vi "5ChPulserTrigs.vi"(1 "Motion Board ID":T3=1 min=1 max=32 step=1, 4 "xmit ring":i32 min=0 max=4 step=1, 5 "mode":T2=enum."Full 25 Ch", 6 "Source":tag="/Dev1/PFI9" caption="Trigger Source", 7 "high time":dbl=5e-06 format="%^.2e", 8 "Axis":T1=1 caption="Axis or Vector Space" items=["Axis 1"=1, "Axis 2"=2, "Axis 3"=3, "Axis 4"=4, "Axis 5"=5, "Axis 6"=6, "Axis 7"=7, "Axis 8"=8, "Vector Space 1"=17, "Vector Space 2"=18, "Vector Space 3"=19, "Vector Space 4"=20], 9 "M-mode?":bool, 10 "error in":errorcluster) -> (0 "5CH Pulser Tasks":refnum<k21>[](array[refnum]), 3 "error out":errorcluster)   [LabVIEW 2022 SP3]
uses:
  ScanningControl/Motion Controllers/-MotionRoutines/MotionGlobals.vi
  <vilib>/DAQmx/configure/trigger.llb/DAQmx Start Trigger (Digital Edge).vi
  <vilib>/DAQmx/create/channels.llb/DAQmx Create Channel (CO-Pulse Generation-Time).vi
  <resource>/objmgr/daqmx.rc
  <vilib>/DAQmx/create/channels.llb/DAQmx Create Channel (CO-Pulse Generation-Frequency).vi
  <vilib>/DAQmx/configure/timing.llb/DAQmx Timing (Implicit).vi
  ScanningControl/Digitizers/-DigitizerRoutines/DigitizerGlobals.vi
  ScanningControl/Switch Modules/SwitchGlobals.vi
  Real Time/-RT_support/RealTimeMode.ctl
  <vilib>/Motion/FlexMotion/CustomControls/CustomControls.llb/AxisOrVectorSpace To Control.flx
panel:
  in  "stop":bool
  # "Counter 1 output is the BNC on grey box."
  # "Trigger source comes from Gate of CTR0 (PFI9)\n\nThe NI trigger connector routes to CTR0 Gate"
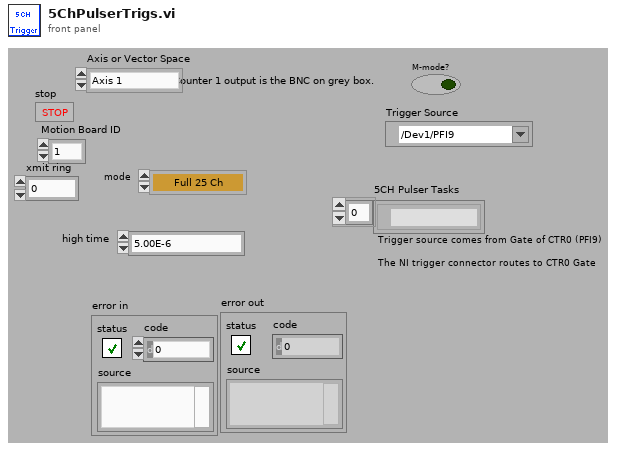
[diagram p1: front panel]
types:
  T1 = typedef "AxisOrVectorSpace To Control.flx" = u16
  T2 = typedef "RealTimeMode.ctl" = enum16{"1T/5R", "1T/5R Deep Mem", "Full 25 Ch", "Drop Ch 5", "Drop Ch 5,4", "Drop Ch 5,4,3", "Drop Ch 5,4,3,2", "All 25 FIFO CH by CH", "Line by line 2 Ch", "Line by line All", "Deep Memory 2 CH", "Drop Ch 5 (3 Trig)", "test", "Drop Ch 5 XMIT", "Drop Ch 5,4 XMIT", "Drop Ch 5,4,3 XMIT"}
  T3 = typedef "Board Id" = u8
  T4 = typedef "DigitizerSettings.ctl" = cluster{"Digitizer delay (us) ":dbl, "rf points per line":i32, "lines per plane":i32, "Samp Rate (Hz)":dbl, "Additional dig delay (us)":dbl, "Voltage Scale":dbl, "Pre-Looks":i32, "Offset delay (us)":dbl, "bits A/D":i8, "Avg Num":i32, "DigTimeOut":sgl, "Rel Dig Delay":sgl, "Dig Ch":i32, "LeCroyCluster":cluster{"LeCroy Channels":bool[], "LC read pt offset":dbl, "Sweep Avg":bool}, "Main Digitizer":T5, "Dig Config":T6, "Digitizer ID Cluster":T7, "Trigger Settings":cluster{"Trig Source":u16, "Trig Coupling":u16, "Trig Slope":u16, "Level (mV)":dbl}, "Bulk Acq":bool, "Bulk Start Indexes":i32[], "Data Ref RF":refnum<data-value>, "NI ID/Channel":cluster{"NI ID":refnum<k15>, "NI CH":i32}[], "Total Dig CH":i32, "Xtra Ann Trig delay (us)":dbl, "Fix Z Delay?":bool, "One Way Transmission?":bool, "Data Ref Log":refnum<data-value>}
  T5 = typedef "Digitizer.ctl" = enum16{"Acqiris Digitizer", "NI Digitizer", "LeCroy", "GaGe", "AlazarTech", "No Digitizer", "Teledyne"}
  T6 = typedef "DigConfig.ctl" = enum16{"Single channel", "2 Chans w/ 2 Acqiris", "2 Chans w/ 1 Acqiris", "5-CH Pulser New", "5-CH pulser w/ ann array", "5-pass style ann array", "Empty"}
  T7 = typedef "DigitizerID.ctl" = cluster{"Acqiris/Alazar/SP ID":u32[], "NI Instr Handles":refnum<k15>[], "LeCroy VISA":refnum<visa-resource-name>, "GaGe Handle":cluster{"Handle":u32, "Sample size":u32, "Resolution":i32, "Offset":i32, "Channels":u32, "Boards":u32}, "ATS Ref":string, "Acqiris Address":string[], "ADQRef":refnum<k24>, "adq_cu_ptr":refnum<k24>}
  T8 = typedef "MotionParameters.ctl" = cluster{"No Motion?":bool, "Motion System":T9, "Motion Bd ID":u8, "Motion Profile":string, "# Axis":i8, "Reverse Z axis?":bool, "SMAC Axis":u16, "scan pair":T10, "RT fps":sgl, "Steps per mm":i32[], "Motor Parameters":cluster{"velocity ct/s":dbl[], "accel ct/s^2":dbl[]}, "One Way Scan":bool, "Reverse One Way Scan":bool, "Global Position (mm)":dbl[], "Plane":i32, "Distance between\nscan lines (um)":sgl, "Distance between\nscan planes (um)":sgl, "number of scan planes":i32, "Total steps in line":i32, "Xtra plane\ndistance  (um)":i32, "Xtra planes ":i32, "Add Axis":bool, "overshoot cts":i32, "BKPT Shift":i32, "Scan Start Time (ms)":u32, "ESP VISA":refnum<visa-resource-name>, "3rd Axis":T11, "GL Ref Out":refnum<k7>, "Galil Address":string}
  T9 = typedef "MotionSys.ctl" = enum16{"MM3000", "NI 735x", "Newport ESP", "No Motion Card", "Galil"}
  T10 = typedef "ScanAxis.ctl" = enum16{"y-(x) scan", "x-(y) scan", "z-(x) scan", "z-(y) scan", "y-(z) scan", "x-(z) scan", "w-(x) scan", "w-(y) scan", "w-(z) scan", "x-(w) scan", "y-(w) scan", "z-(w) scan"}
  T11 = typedef "3rdAxis.ctl" = u16
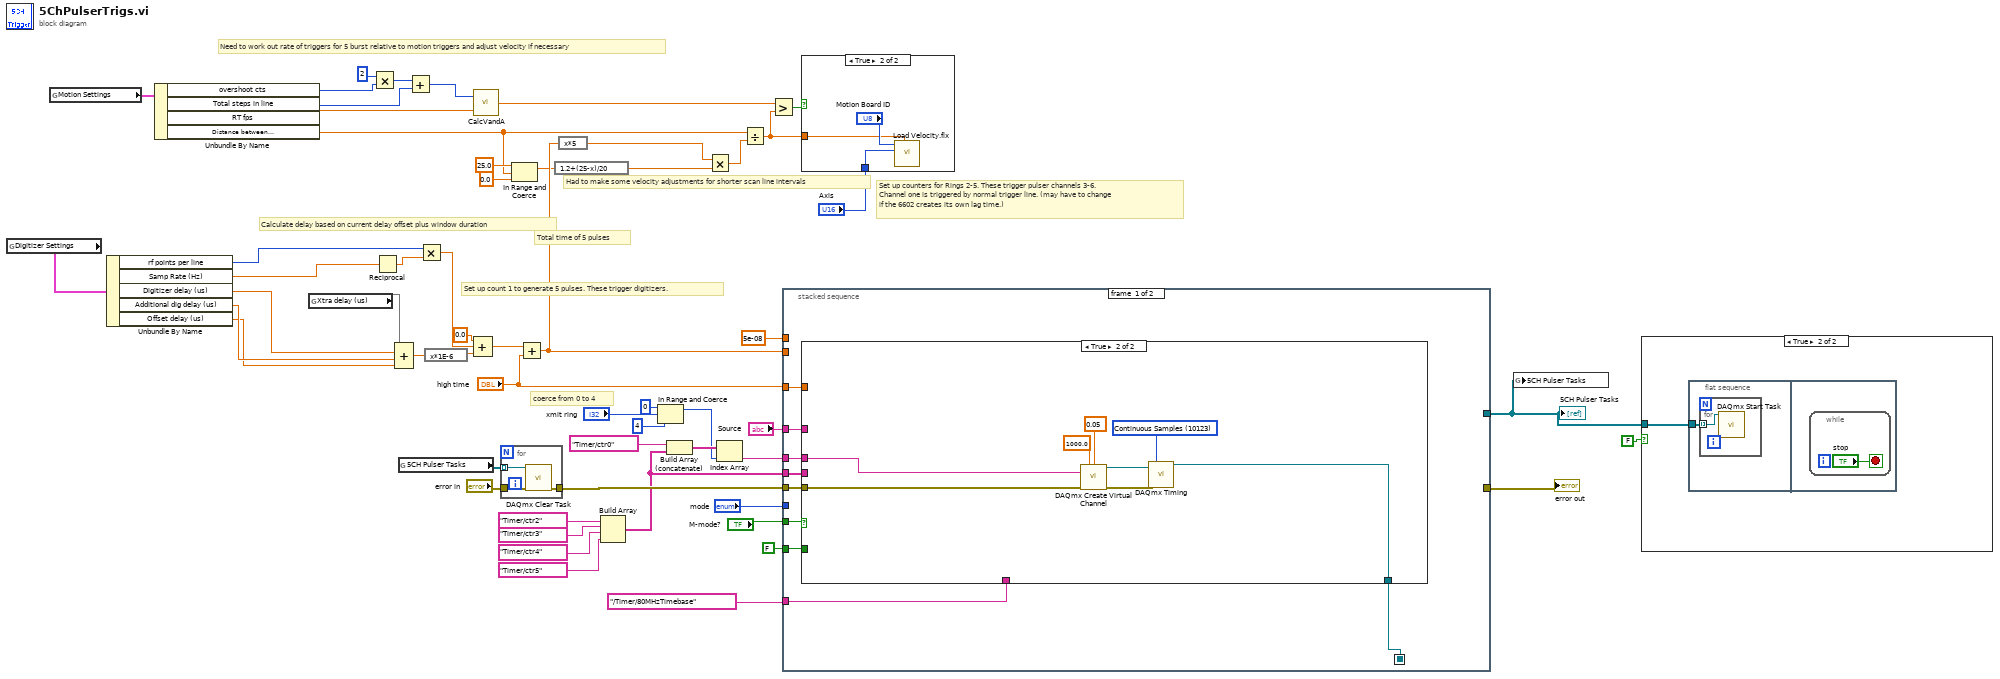
[diagram p0: block diagram]
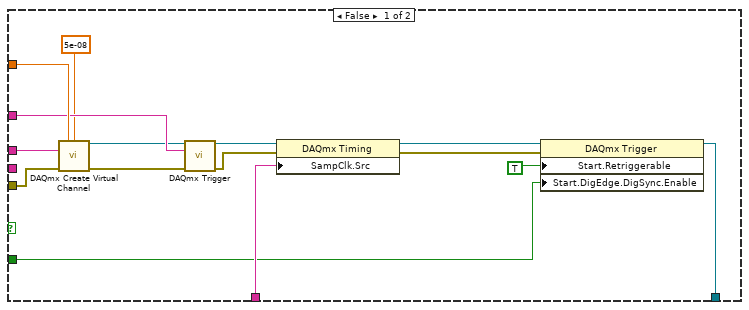
[diagram p2: hidden frame]
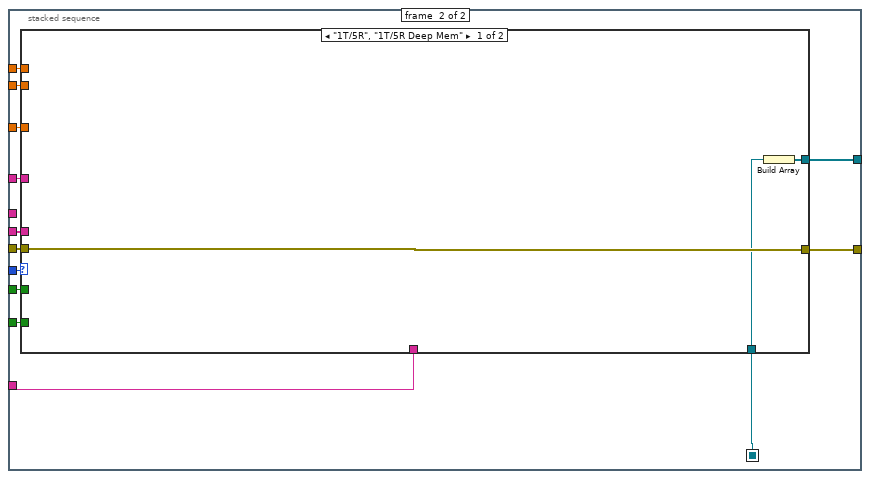
[diagram p3: hidden frame]
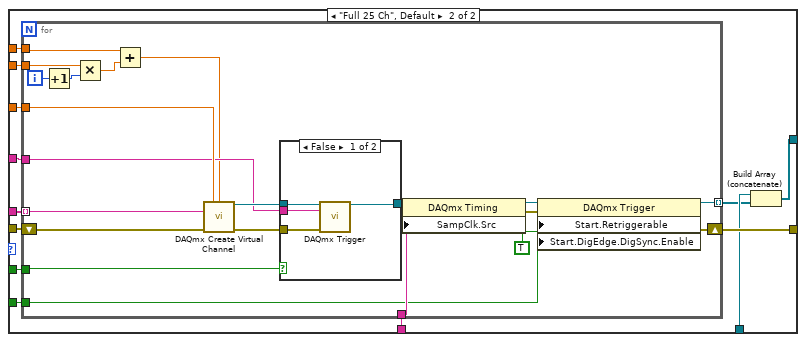
[diagram p4: hidden frame]
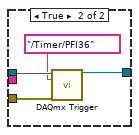
[diagram p5: hidden frame]
diagram:
  # "coerce from 0 to 4"
  # "Had to make some velocity adjustments for shorter scan line intervals"
  # "Total time of 5 pulses"
  # "Need to work out rate of triggers for 5 burst relative to motion triggers and adjust velocity if necessary"
  # "Set up counters for Rings 2-5. These trigger pulser channels 3-6.\nChannel one is triggered by normal trigger line. (may have to change \nif the 6602 creates its own lag time.)"
  # "Set up count 1 to generate 5 pulses. These trigger digitizers."
  # "Calculate delay based on current delay offset plus window duration"
  n1 = global read "DigitizerGlobals.vi" "Digitizer Settings"() -> (w7:T4)
  n2 = global read "MotionGlobals.vi" "Motion Settings"() -> (w12:T8)
  n3 = Unbundle By Name(w7) -> ("rf points per line"=w6:i32, "Samp Rate (Hz)"=w5:dbl, "Digitizer delay (us)"=w3:dbl, "Additional dig delay (us)"=w2:dbl, "Offset delay (us)"=w1:dbl)
  n4 = Unbundle By Name(w12) -> ("overshoot cts"=w11:i32, "Total steps in line"=w10:i32, "RT fps"=w9:sgl, "Distance between\nscan lines (um)"=w8:sgl)
  n5 = global read "SwitchGlobals.vi" "Xtra delay (us)"() -> (w4)
  n6 = Multiply(x=2, y=w11) -> (x*y=w45:i32)
  n7 = Reciprocal(x=w5) -> (1/x=w56:dbl)
  n8 = Compound Arithmetic op=ADD(w4, w3, w2, w1) -> (w29:dbl)
  n9 = global read "MotionGlobals.vi" "5CH Pulser Tasks"() -> (w51:refnum<k21>[])
  n10 = Add(x=w45, y=w10) -> (x+y=w44:i32)
  n11 = Multiply(x=w6, y=w56) -> (x*y=w57:dbl)
  n12 = expression code="x*1E-6"(w29) -> (w28:dbl)
  n13 = call "CalcVandA.vi"("distance"=w44, "fps"=w9) -> ("Velocity"=w42:dbl)  [unwired: 2 out]
  n14 = Compound Arithmetic op=ADD(0.0 ("y"), w57, w28) -> (w38:dbl)
  n15 = for {
    tunnel: [w60] -> w39
    tunnel: w51 -> [w59] mode=indexing
    tunnel: "error in" -> [w58]
    n16 = call <vilib>:"DAQmx Clear Task.vi"("task in"=w59, "error in"=w58) -> ("error out"=w60:errorcluster)  [unwired: 13 out]
  }
  n17 = In Range and Coerce(upper limit=sgl 25.0, x=w8, lower limit=sgl 0.0) -> (coerced(x)=w37:sgl)  [unwired: 1 out]
  n18 = Add(x=w38, y="high time") -> (x+y=w43:dbl)
  n19 = expression code="1.2+(25-x)/20"(w37) -> (w34:sgl)
  n20 = expression code="x*5"(w43) -> (w33:dbl)
  n21 = Build Array(tag "Timer/ctr2" ("Counter(s)"), tag "Timer/ctr3" ("Counter(s)"), tag "Timer/ctr4" ("Counter(s)"), tag "Timer/ctr5" ("Counter(s)")) -> (w21:tag[])
  n22 = In Range and Coerce(upper limit=0, x="xmit ring", lower limit=4) -> (coerced(x)=w14:i32)  [unwired: 1 out]
  n23 = Build Array (concatenate)(tag "Timer/ctr0" ("Counter(s)"), w21) -> (w19:tag[])
  n24 = Multiply(x=w33, y=w34) -> (x*y=w32:dbl)
  n25 = Index Array(array=w19, index=w14) -> (element=w18:tag)
  n26 = Divide(x=w8, y=w32) -> (x/y=w40:dbl)
  n27 = Greater?(x=w42, y=w40) -> (0:w41:bool)
  n28 = stacked-sequence {
    seq-local: [w63 _] -> [_ w96]
    tunnel: [_ w105] -> w53
    tunnel: "Source" -> [w67 w104]
    tunnel: w39 -> [w69 w103]
    tunnel: "high time" -> [w68 w102]
    tunnel: w21 -> [w61 w101]
    tunnel: w43 -> [_ w100]
    tunnel: "mode" -> [_ w99]
    tunnel: tag "/Timer/80MHzTimebase" ("SampClk.Src") -> [w66 w98]
    tunnel: FALSE -> [w65 w97]
    tunnel: w18 -> [w64 _]
    tunnel: [_ w95] -> w23
    tunnel: "M-mode?" -> [w62 w94]
    tunnel: 5e-08 ("x") -> [_ w93]
    frame #0 {
      n29 = case shown="True" w62 {
        tunnel: w69 -> [w84 w92]
        tunnel: w68 -> [w83 _]
        tunnel: w67 -> [w82 _]
        tunnel: w66 -> [w81 _]
        tunnel: w65 -> [w80 _]
        tunnel: w64 -> [w72 w85]
        tunnel: [w71 w86] -> w63
        tunnel: w61 -> [_ _]
        frame False {
          n30 = call-poly <vilib>:"DAQmx Create Virtual Channel.vi"("high time"=w83, "low time"=5e-08 ("x"), "counter"=w72, "error in"=w84) -> ("task out"=w78:refnum<k21>, "error out"=w77:errorcluster)  [unwired: 5 in, 5 out]
          n31 = call-poly <vilib>:"DAQmx Trigger.vi"("task/channels in"=w78, "source"=w82, "error in"=w77) -> ("task out"=w76:refnum<k21>, "error out"=w70:errorcluster)  [unwired: 1 in, 10 out]
          n32 = property class="DAQmx Timing"(reference=w76, error in=w70, "SampClk.Src"=w81) -> (reference out=w75:refnum<k21>, error out=w74:errorcluster)
          n33 = property class="DAQmx Trigger"(reference=w75, error in=w74, "Start.Retriggerable"=TRUE, "Start.DigEdge.DigSync.Enable"=w80) -> (reference out=w71:refnum<k21>)  [unwired: 1 out]
        }
        frame True {
          w89 = 10123 items=["Finite Samples"=10178, "Continuous Samples"=10123, "Hardware Timed Single Point"=12522] ("sample mode")
          n34 = call-poly <vilib>:"DAQmx Create Virtual Channel.vi"("frequency"=1000.0, "duty cycle"=0.05, "counter"=w85, "error in"=w92) -> ("task out"=w88:refnum<k21>, "error out"=w87:errorcluster)  [unwired: 5 in, 5 out]
          n35 = call-poly <vilib>:"DAQmx Timing.vi"("task/channels in"=w88, "sample mode"=w89, "error in"=w87) -> ("task out"=w86:refnum<k21>)  [unwired: 11 in, 1 out]
        }
      }
    }
    frame #1 {
      n36 = case shown="\"1T/5R\", \"1T/5R Deep Mem\"" w99 {
        tunnel: [w108 w121] -> w105
        tunnel: w104 -> [_ w120]
        tunnel: w103 -> [w108 w119]
        tunnel: w102 -> [_ w118]
        tunnel: w101 -> [_ w117]
        tunnel: w100 -> [_ w116]
        tunnel: w98 -> [_ w115]
        tunnel: w97 -> [_ w114]
        tunnel: w96 -> [w107 w113]
        tunnel: [w106 w111] -> w95
        tunnel: w94 -> [_ w110]
        tunnel: w93 -> [_ w109]
        frame "1T/5R", "1T/5R Deep Mem" {
          n37 = Build Array(w107) -> (w106:refnum<k21>[])
        }
        frame "Full 25 Ch", Default {
          n38 = for {
            tunnel: w116 -> [w141]
            tunnel: w118 -> [w133]
            shift-right: [w137] -> w121
            shift-left: w119 -> [w140]
            tunnel: w109 -> [w132]
            tunnel: w120 -> [w126]
            tunnel: w117 -> [w136] mode=indexing
            tunnel: w115 -> [w127]
            tunnel: w114 -> [w125]
            tunnel: [w124] -> w112 mode=indexing
            tunnel: w110 -> [w123]
            i -> [w142]
            n39 = Increment(x=w142) -> (x+1=w135:i32)
            n40 = Multiply(x=w141, y=w135) -> (x*y=w139:dbl)
            n41 = Add(x=w132, y=w139) -> (x+y=w122:dbl)
            n42 = call-poly <vilib>:"DAQmx Create Virtual Channel.vi"("high time"=w133, "low time"=w122, "counter"=w136, "error in"=w140) -> ("task out"=w134:refnum<k21>, "error out"=w138:errorcluster)  [unwired: 5 in, 5 out]
            n43 = case shown="False" w123 {
              tunnel: w138 -> [w145 w150]
              tunnel: w134 -> [w146 w149]
              tunnel: [w144 w148] -> w128
              tunnel: w126 -> [w143 _]
              frame False {
                n44 = call-poly <vilib>:"DAQmx Trigger.vi"("task/channels in"=w146, "source"=w143, "error in"=w145) -> ("task out"=w144:refnum<k21>)  [unwired: 2 in, 10 out]
              }
              frame True {
                n45 = call-poly <vilib>:"DAQmx Trigger.vi"("task/channels in"=w149, "source"=tag "/Timer/PFI36", "error in"=w150) -> ("task out"=w148:refnum<k21>)  [unwired: 1 in, 11 out]
              }
            }
            n46 = property class="DAQmx Timing"(reference=w128, "SampClk.Src"=w127) -> (reference out=w131:refnum<k21>, error out=w129:errorcluster)  [unwired: 1 in]
            n47 = property class="DAQmx Trigger"(reference=w131, error in=w129, "Start.Retriggerable"=TRUE, "Start.DigEdge.DigSync.Enable"=w125) -> (reference out=w124:refnum<k21>, error out=w137:errorcluster)
          }
          n48 = Build Array (concatenate)(w113, w112) -> (w111:refnum<k21>[])
        }
      }
    }
  }
  "error out" <- w53
  "5CH Pulser Tasks" <- w23
  n49 = case shown="True" w41 {
    tunnel: w40 -> [_ w152]
    tunnel: "Axis" -> [_ w151]
    frame False {
    }
    frame True {
      n50 = call <vilib>:"Load Velocity.flx"("Velocity (10000)"=w152, "Axis or Vector Space"=w151, "Board ID"="Motion Board ID") -> ()  [unwired: 1 in, 6 out]
    }
  }
  n51 = global write "MotionGlobals.vi" "5CH Pulser Tasks"(w23) -> ()
  n52 = case shown="True" FALSE {
    tunnel: w23 -> [_ w154]
    frame False {
    }
    frame True {
      n53 = flat-sequence {
        tunnel: w154 -> [w155]
        frame #0 {
          n54 = for {
            tunnel: w155 -> [w156] mode=indexing
            n55 = call <vilib>:"DAQmx Start Task.vi"("task/channels in"=w156) -> ()  [unwired: 13 in, 2 out]
          }
        }
        frame #1 {
          n56 = while {
            stop <- "stop" stop-if-true
          }
        }
      }
    }
  }
